vi "Block Profile Measurement v3.vi"() -> ()   [LabVIEW 2011]
uses:
  <vilib>/Utility/error.llb/DialogType.ctl
  <vilib>/DAQmx/read.llb/DAQmx Read (Analog 1D DBL NChan 1Samp).vi
  <vilib>/DAQmx/create/channels.llb/DAQmx Create Channel (AI-Current-Basic).vi
  <vilib>/DAQmx/configure/timing.llb/DAQmx Timing.vi
  <vilib>/DAQmx/configure/trigger.llb/DAQmx Start Trigger (Analog Edge).vi
  <vilib>/DAQmx/miscellaneous.llb/DAQmx Fill In Error Info.vi
  <vilib>/Analysis/NI_AALBase.lvlib
panel:
  in  "Level":dbl=0.5 format="%0.2f"
  in  "Slope":i32(ring)=10280 items=["Rising"=10280, "Falling"=10171]
  in  "Source":string="PFI0" caption="Trigger Source*"
  in  "stop":bool
  out "Measurement":waveform(dbl)[](graph)
  in  "Maximum Value":dbl=10.0 format="%0.2f"
  in  "Minimum Value":dbl=-10.0 format="%0.2f"
  in  "Rate":dbl=50000.0 caption="Sample Rate (Hz)" format="%0.2f"
  in  "Samples per Channel":i32=2048
  in  "Physical Channel":tag="Dev1/ai0"
  out "Scaled Values":dbl[](array[numeric])=[0.0, 1.0] format="%.3p"
  out "Measurements / Block":i32
  in  "ECOLAB Button":bool
  out "Maximum":string="0.000"
  out "Block Count":i32
  in  "Tab Control":enum32{"DISPLAY", "CONFIG", "CALIBRATE"}(tab)
  in  "Intervals":i32=20
  out "XY Graph":cluster{dbl[], "Initialize Value":dbl[]}[](graph)
  out "Histogram Graph":T1(graph)={"X Values"=[0.0, 0.0, 0.0, 0.0, 0.0, 0.0, 0.0, 0.0, 0.0, 0.0, 0.0, 0.0, 0.0, 0.0, 0.0, 0.0, 0.0, 0.0, 0.0, 0.0], "Histogram: h(x)"=[0, 0, 0, 0, 0, 0, 0, 0, 0, 0, 0, 0, 0, 0, 0, 0, 0, 0, 0, 1]}
  in  "Thresh Compare 2":bool=TRUE
  in  "Threshold Value SP 2":dbl=0.004
  in  "Thresh Compare":bool=TRUE
  out "Save Error":errorcluster
  out "Main Error":errorcluster
  out "DAQ Error":errorcluster={"status"=TRUE, "code"=-200478, "source"="Block Profile Measurement v3.vi<append>\n<B>Task Name: </B>mA"}
  in  "DAQ Selection":tag="cDAQ1Mod1/ai0:1"
  in  "Comments (Saves to Data File)":string
  out "DAQ Loop":i32=1641
  out "File Path Output":path=path "H:/Projects/Chris Opelt/Data Files/Data-1-23-2012-{9-AM}.xls"
  in  "Maximum Array Size":i32=200
  in  "Threshold Value SP":dbl=0.004
  in  "DAQ wait ms":u32=1
  in  "Scale":T2={"Channel Select"=0, "Clear/Reset Scales"=FALSE, "Channel #"=["0", "1"], "Scale Names"=["Laser", "Ultra-Sonic"], "Set?"=[FALSE, FALSE, FALSE, FALSE], "HI/LO Setpoints"=[1.0, 0.0, 1.0, 0.0], "Units"=["inches", "inches"], "HI/LO Signals"=[0.02, 0.004, 0.02, 0.004], "Slope/Intercept"=[1.0, 0.0, 1.0, 0.0], "IN/OUT Values"=[0.0, 0.0, 1.0, 1.0], "Sim Signals?"=FALSE, "Sim. Signal"=0.0} {"Sim. Signal" format="%#.3p"; "Channel Select" min=0 step=1; "Slope/Intercept" format="%#.3p"; "HI/LO Setpoints" format="%#.3p"; "IN/OUT Values" format="%#.3p"; "HI/LO Signals" format="%#.3p"}
  in  "Stop Program":bool=TRUE
  in  "Reset Block Count?":bool
  # "Maximum (inches)"
  # "Measurements/Block"
  # "Laser"
  # "Ultrasonic"
  # "Block Count"
  # "Block Profile Measurement Program"
  # "Blake Otting - 2011"
  # "Histogram of Maximum Value Measurements"
  # "Measurement Profile of Last Block"
  # "Laser and Ultrasonic measurements are half-sampled before saving to data row.\nLaser and Ultrasonic measurements are separated by an asterisk in the data row."
  # "Histogram represents laser measurements"
  # "Laser Specs:\nRange:  1.8\" to 2.4\"\nFocal Point:  2.8\"\nResolution:  0.0001\" @ 50mm\nSignal: 4 to 20mA"
  # "These settings should be OK"
  # "Threshold Settings\n(Block Detection & Data Logging Trigger)"
  # "Ultrasonic Specs:\nRange:  1.2\" to 11.8\"\nResolution:  0.025\"\nSignal: 4 to 20mA"
  # "Comparison"
  # "Setpoint (inches)"
  # "LASER"
  # "Comparison"
  # "Setpoint (inches)"
  # "Set to Range (both):\n1.85\" and 2.35\""
  # "ULTRASONIC"
  # "Ch.\n#"
  # "Scale\nName"
  # "Set\nValues?"
  # "Channel\nSelect"
  # "Scaled"
  # "Pre-Scaled"
  # "Scaling Result"
  # "Values"
  # "Units"
  # "Values"
  # "HI"
  # "Slope"
  # "IN"
  # "LO"
  # "Intercept"
  # "OUT"
  # "HI"
  # "Slope"
  # "IN"
  # "LO"
  # "Intercept"
  # "OUT"
  # "HI"
  # "Slope"
  # "IN"
  # "LO"
  # "Intercept"
  # "OUT"
  # "HI"
  # "Slope"
  # "IN"
  # "LO"
  # "Intercept"
  # "OUT"
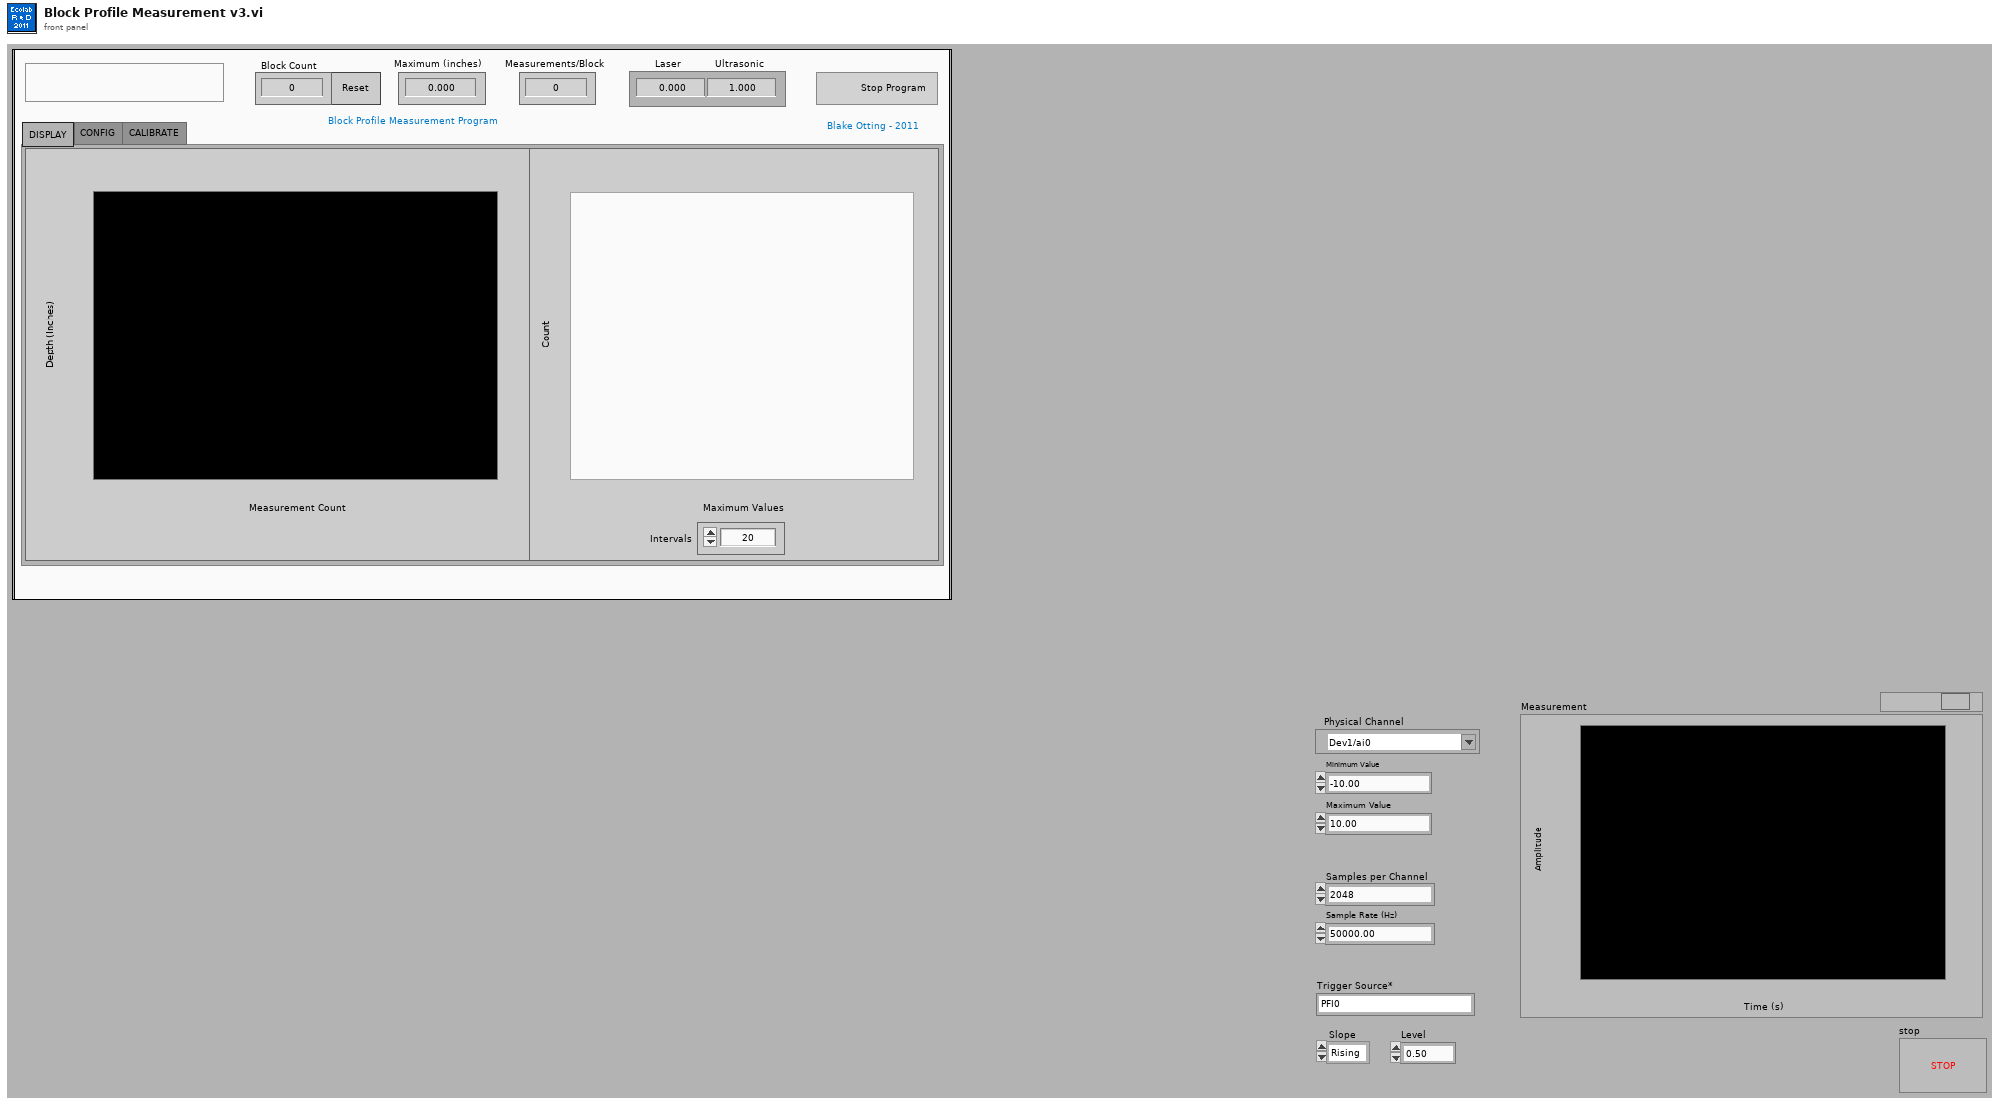
[diagram p1: front panel]
types:
  T1 = cluster{"X Values":dbl[], "Histogram: h(x)":i32[]}
  T2 = cluster{"Channel Select":i32, "Clear/Reset Scales":bool, "Channel #":string[], "Scale Names":string[], "Set?":bool[], "HI/LO Setpoints":dbl[], "Units":string[], "HI/LO Signals":dbl[], "Slope/Intercept":dbl[], "IN/OUT Values":dbl[], "Sim Signals?":bool, "Sim. Signal":dbl}
  T3 = typedef "DialogType.ctl" = u16
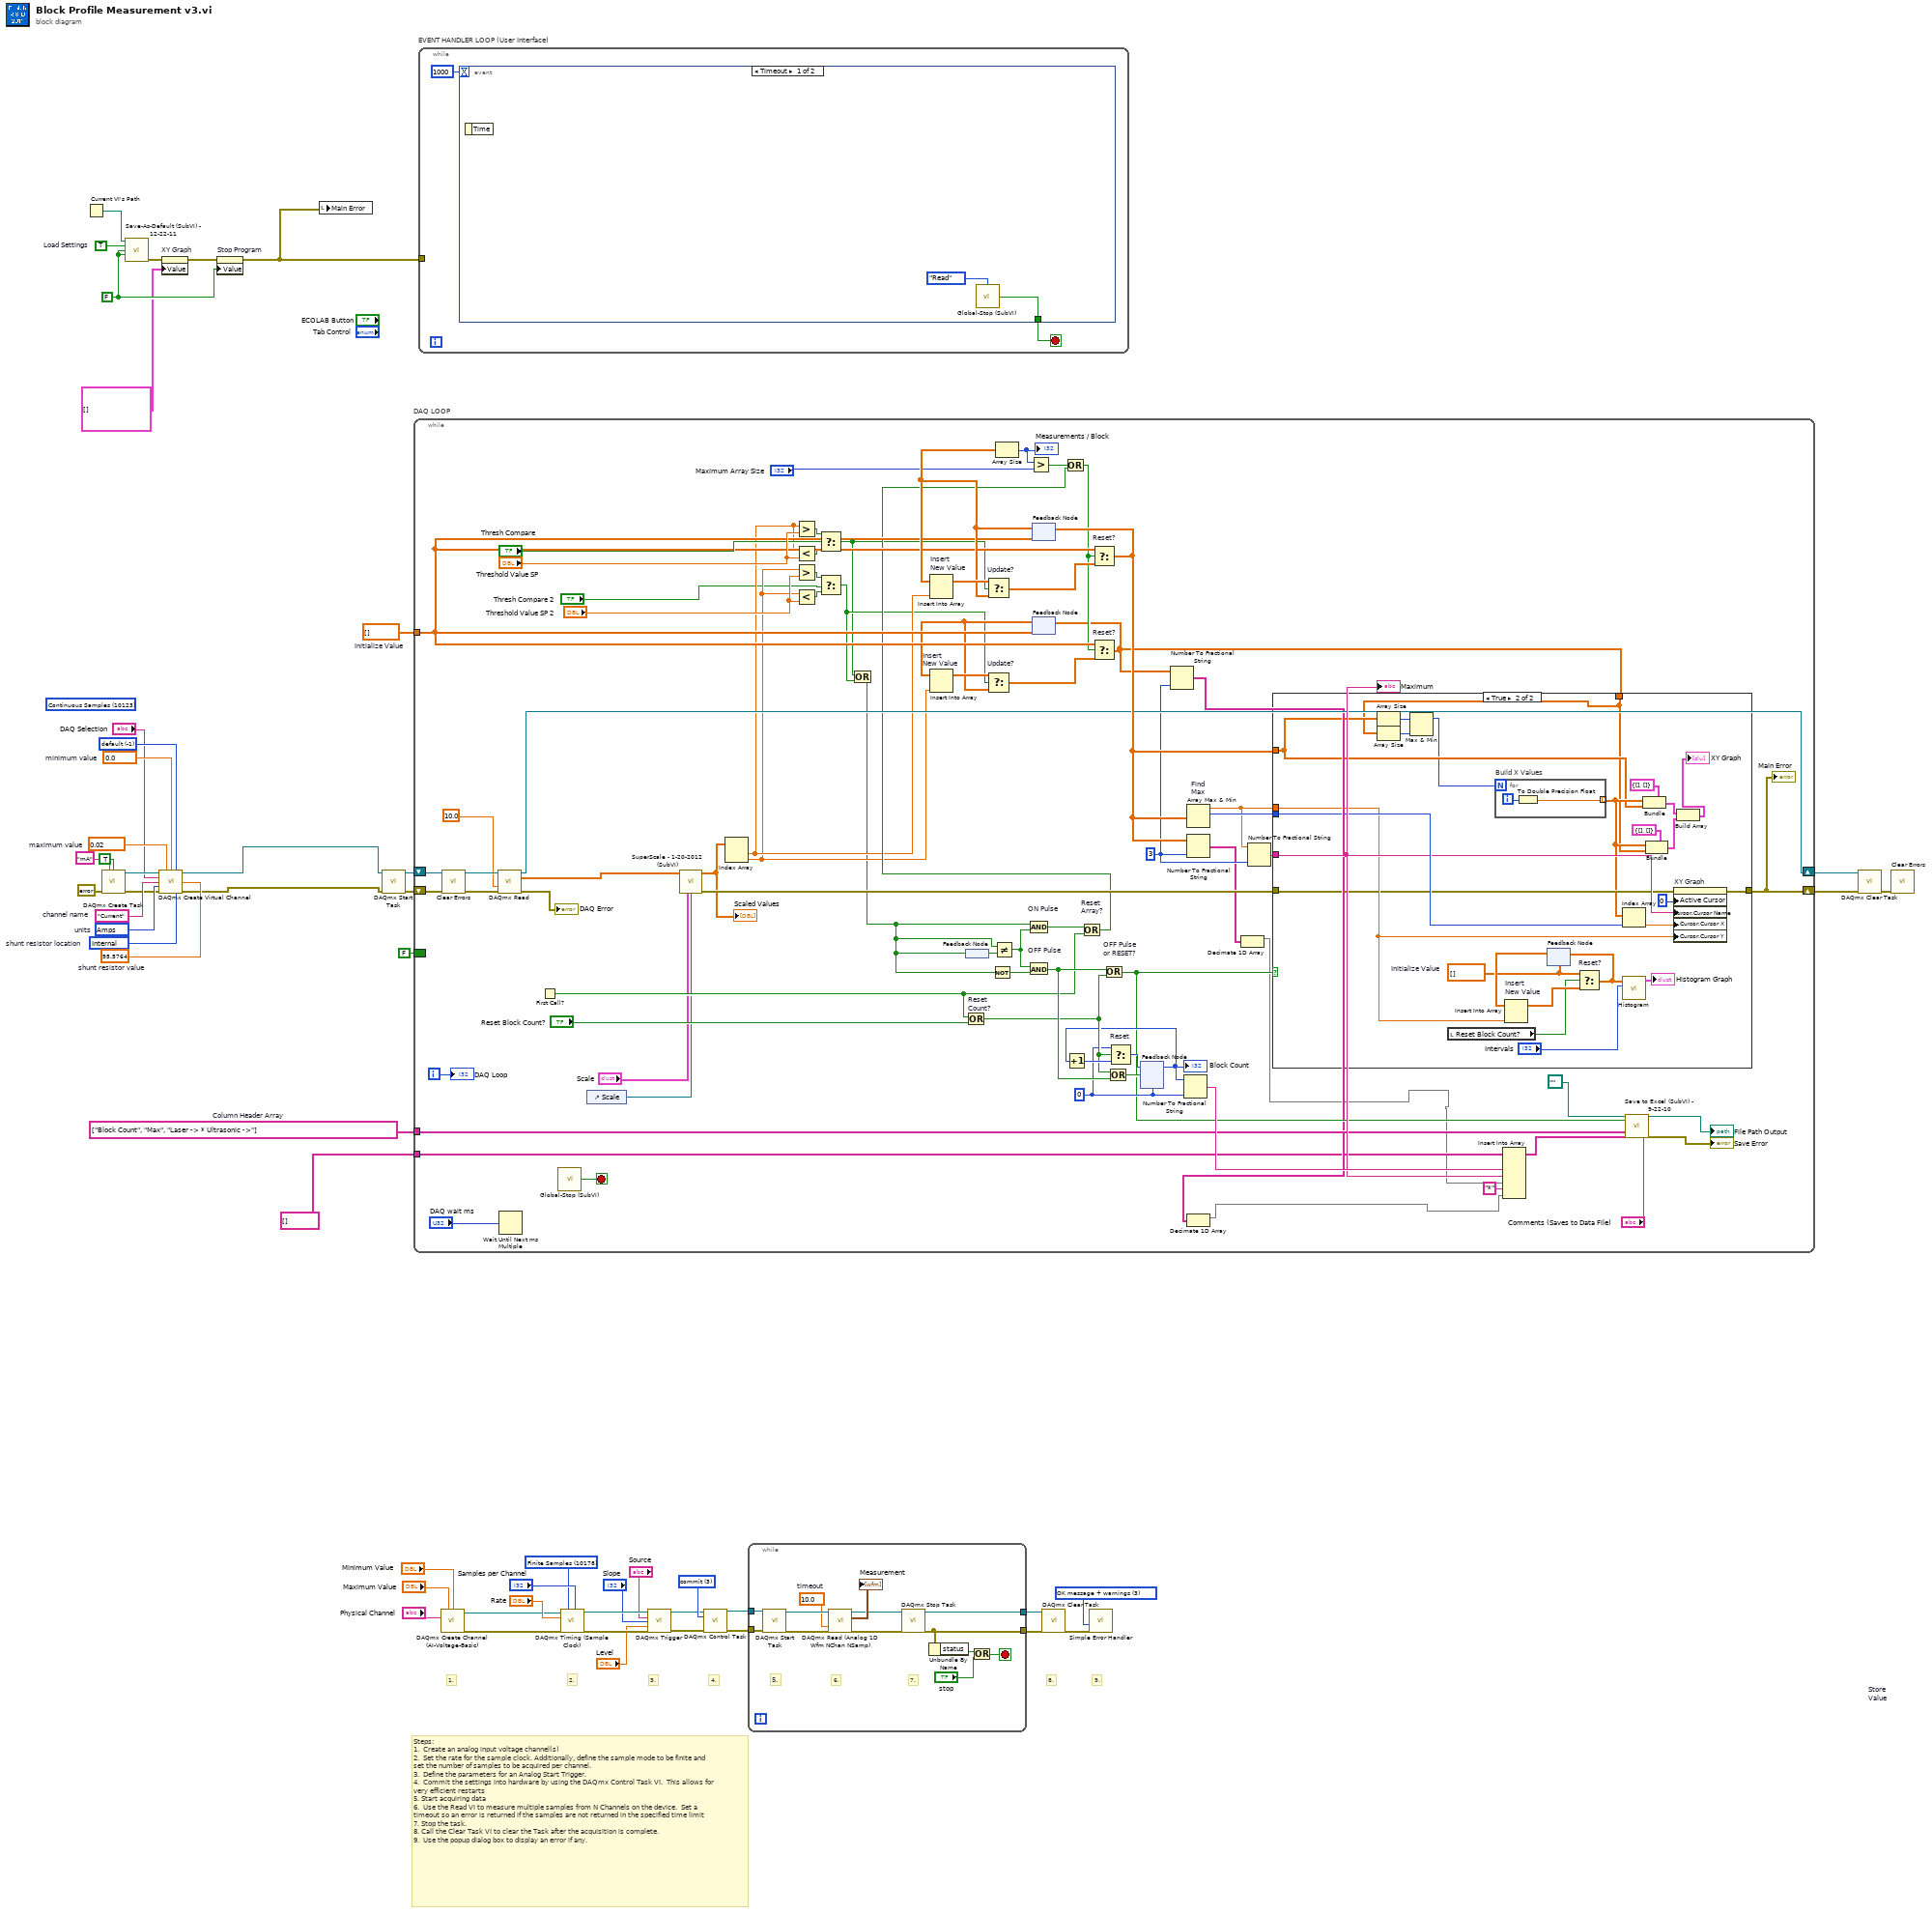
[diagram p0: block diagram]
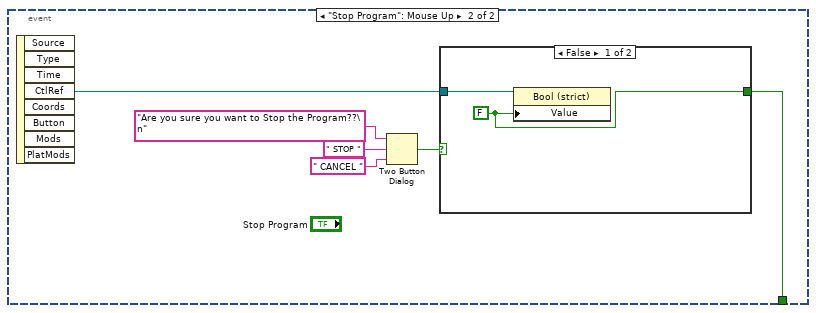
[diagram p2: hidden frame]
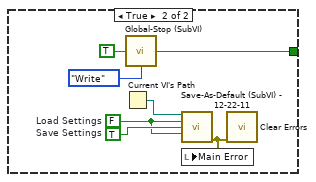
[diagram p3: hidden frame]
diagram:
  w12 = 3 items=["verify"=2, "reserve"=4, "commit"=3, "unreserve"=5, "abort"=6] ("action")
  w13 = T3 3 items=["no dialog", "OK message", "continue or stop message", "OK message + warnings", "continue/stop + warnings"] ("type of dialog (OK msg:1)")
  w14 = 10178 items=["Finite Samples"=10178, "Continuous Samples"=10123] ("sample mode")
  w32 = string[] ["Block Count", "Max", "Laser -> * Ultrasonic ->"]  # Column Header Array
  w34 = dbl[] []  # Initialize Value
  w38 = TRUE  # Load Settings
  w37 = FALSE
  (unwired) 10123 items=["Finite Samples"=10178, "Continuous Samples"=10123, "Hardware Timed Single Point"=12522] ("Sample Mode")
  w46 = -1 items=["default"=-1, "RSE"=10083, "NRSE"=10078, "Differential"=10106, "Pseudodifferential"=12529]
  w47 = 10342 items=["Amps"=10342, "From Custom Scale"=10065]  # units
  w48 = 95.5764  # shunt resistor value
  w49 = 10200 items=["Internal"=10200, "External"=10167]  # shunt resistor location
  w50 = "Current"  # channel name
  w51 = 0.0  # minimum value
  w52 = 0.02  # maximum value
  # "9."
  # "8."
  # "4."
  # "Steps: \n1.  Create an analog input voltage channel(s)\n2.  Set the rate for the sample clock. Additionally, define the sample mode to be finite and set the number of samples to be acquired per channel.\n3.  Define the parameters for an Analog Start Trigger.\n4.  Commit the settings into hardware by using the DAQmx Control Task VI.  This allows for very efficient restarts\n5. Start acquiring data\n6.  Use the Read VI to measure multiple samples from N Channels on the device.  Set a timeout so an error is returned if the samples are not returned in the specified time limit\n7. Stop the task.\n8. Call the Clear Task VI to clear the Task after the acquisition is complete.\n9.  Use the popup dialog box to display an error if any."
  # "3."
  # "2."
  # "1."
  n1 = Current VI's Path() -> (path=w39:path)
  n2 = call <vilib>:"DAQmx Create Task.vi"("new task name"="mA", "auto cleanup"=TRUE, "error in"=errorcluster {"status"=FALSE, "code"=0, "source"=""}) -> ("task out"=w45:refnum<k21>, "error out"=w44:errorcluster)  [unwired: 11 in]
  n3 = call "Save-As-Default (SubVI) - 12-22-11.vi"("Current VI's Path"=w39, "Load Settings"=w38, "Save Settings"=w37, "Save and Exit"=w37) -> ("Error Output"=w36:errorcluster)  [unwired: 11 in]
  n4 = call-poly <vilib>:"DAQmx Create Virtual Channel.vi"("task in"=w45, "maximum value"=w52, "minimum value"=w51, "input terminal configuration"=w46, "physical channels"="DAQ Selection", "name to assign"=w50, "external shunt resistor value"=w48, "units"=w47, "error in"=w44, "shunt resistor location"=w49) -> ("task out"=w24:refnum<k21>, "error out"=w23:errorcluster)  [unwired: 1 in, 3 out]
  n5 = property on="XY Graph" class="XYGraph (strict)"(error in=w36, "Value"=cluster{dbl[], "Initialize Value":dbl[]}[] [] ("XY Graph")) -> (error out=w35:errorcluster)  [unwired: 1 in, 1 out]
  n6 = property on="Stop Program" class="Bool (strict)"(error in=w35, "Value"=w37) -> (error out=w33:errorcluster)  [unwired: 1 in, 1 out]
  n7 = local write "Main Error"(w33) -> ()
  n8 = call <vilib>:"DAQmx Start Task.vi"("task/channels in"=w24, "error in"=w23) -> ("task out"=w29:refnum<k21>, "error out"=w27:errorcluster)  [unwired: 12 in]
  n9 = while "DAQ LOOP" {
    tunnel: w34 -> [w82]
    tunnel: w32 -> [w102]
    tunnel: string[] [] ("F-format string") -> [w76]
    shift-right: [w94] -> w28
    shift-left: w29 -> [w90]
    shift-right: [w97] -> w40
    shift-left: w27 -> [w91]
    border: FALSE -> [_]
    i -> [w126]
    stop <- w124 stop-if-true
    w79 = i16 3 ("precision (6)")
    w99 = 0 ("index")
    n10 = call <vilib>:"Clear Errors.vi"("error in (no error)"=w91) -> ("error out"=w89:errorcluster)  [unwired: 6 in]
    n11 = call-poly <vilib>:"DAQmx Read.vi"("task/channels in"=w90, "timeout"=10.0, "error in"=w89) -> ("task out"=w94:refnum<k21>, "data"=w54:dbl[], "error out"=→"DAQ Error":errorcluster)  [unwired: 10 in]
    n12 = Wait Until Next ms Multiple(millisecond multiple="DAQ wait ms") -> ()  [unwired: 1 out]
    n13 = First Call?() -> (First Call?: T/F=w100:bool)
    n14 = call "Global-Stop (SubVI).vi"() -> ("OUT"=w124:bool)  [unwired: 4 in]
    n15 = control-ref of="Scale"() -> (w69:refnum<vi>)
    n16 = call "SuperScale - 1-20-2012 (SubVI).vi"("Measured Signals"=w54, "Scale Template"="Scale", "Scale Reference"=w69) -> ("Scaled Values"=w66:dbl[], "Scale Error"=w98:errorcluster)  [unwired: 11 in]
    "Scaled Values" <- w66
    n17 = Index Array(array=w66) -> (element #1=w61:dbl, element #2=w60:dbl)  [unwired: 2 in]
    n18 = Greater?(x=w61, y="Threshold Value SP") -> (0:w68:bool)
    n19 = Less?(x=w61, y="Threshold Value SP") -> (x < y?=w67:bool)
    n20 = Greater?(x=w60, y="Threshold Value SP 2") -> (0:w64:bool)
    n21 = Less?(x=w60, y="Threshold Value SP 2") -> (x < y?=w63:bool)
    n22 = Select(t=w68, s="Thresh Compare", f=w67) -> (s? t:f=w57:bool)
    n23 = Select(t=w64, s="Thresh Compare 2", f=w63) -> (s? t:f=w58:bool)
    n24 = Or(x=w57, y=w58) -> (x .or. y?=w56:bool)
    n25 = Or "Reset\nCount?"(x=w100, y="Reset Block Count?") -> (x .or. y?=w114:bool)
    n26 = feedback #1() -> (w121:bool)
    n27 = feedback-in #1(w56) -> ()
    n28 = Not(x=w56) -> (.not. x?=w119:bool)
    n29 = Not Equal?(x=w56, y=w121) -> (x != y?=w120:bool)
    n30 = And "ON Pulse"(x=w56, y=w120) -> (x .and. y?=w101:bool)
    n31 = And "OFF Pulse"(x=w120, y=w119) -> (x .and. y?=w115:bool)
    n32 = feedback #2(w82) -> (w88:dbl[])
    n33 = Insert Into Array "Insert \nNew Value"(array=w88, new element=w61) -> (w123:dbl[])  [unwired: 1 in]
    n34 = Select "Update?"(t=w123, s=w57, f=w88) -> (s? t:f=w122:dbl[])
    n35 = Array Size(array=w88) -> (size(s)=w87:i32)
    "Measurements / Block" <- w87
    n36 = Greater?(x=w87, y="Maximum Array Size") -> (0:w85:bool)
    n37 = feedback #3(w82) -> (w80:dbl[])
    n38 = Insert Into Array "Insert \nNew Value"(array=w80, new element=w60) -> (w84:dbl[])  [unwired: 1 in]
    n39 = Select "Update?"(t=w84, s=w58, f=w80) -> (s? t:f=w83:dbl[])
    n40 = Or "Reset\nArray?"(x=w101, y=w100) -> (x .or. y?=w72:bool)
    n41 = Or(x=w85, y=w72) -> (x .or. y?=w81:bool)
    n42 = Select "Reset?"(t=w82, s=w81, f=w122) -> (s? t:f=w103:dbl[])
    n43 = feedback-in #2(w103) -> ()
    n44 = Select "Reset?"(t=w82, s=w81, f=w83) -> (s? t:f=w71:dbl[])
    n45 = feedback-in #3(w71) -> ()
    n46 = Or "OFF Pulse\nor RESET?"(x=w115, y=w114) -> (x .or. y?=w95:bool)
    n47 = Or(x=w114, y=w115) -> (x .or. y?=w116:bool)
    n48 = feedback #4 "Store\nValue"(w99) -> (w107:i32)
    "Block Count" <- w107
    n49 = Increment(x=w107) -> (x+1=w118:i32)
    n50 = Select "Reset"(t=w99, s=w114, f=w118) -> (s? t:f=w117:i32)
    n51 = feedback-in #4(w117, w116) -> ()
    n52 = Number To Fractional String(number=w71, precision (6)=w79) -> (F-format string=w78:string[])  [unwired: 2 in]
    n53 = Number To Fractional String(number=w107, precision (6)=w99) -> (F-format string=w112:string)  [unwired: 2 in]
    n54 = Decimate 1D Array(w78) -> (w73:string[])  [unwired: 1 out]
    n55 = Array Max & Min "Find\nMax"(array=w103) -> (max value=w105:dbl, max index (indices)=w106:i32)  [unwired: 2 out]
    n56 = Number To Fractional String(number=w103, precision (6)=w79) -> (F-format string=w77:string[])  [unwired: 2 in]
    n57 = Decimate 1D Array(w77) -> (w74:string[])  [unwired: 1 out]
    n58 = Number To Fractional String(number=w105, precision (6)=w79) -> (F-format string=w104:string)  [unwired: 2 in]
    "Maximum" <- w104
    n59 = case shown="True" w95 {
      tunnel: w103 -> [_ w132]
      tunnel: w106 -> [_ w144]
      tunnel: w104 -> [_ w143]
      tunnel: w105 -> [_ w142]
      tunnel: w98 -> [w127 w139]
      tunnel: [w127 w138] -> w97
      tunnel: w71 -> [_ w130]
      frame False {
      }
      frame True {
        w151 = dbl[] []  # Initialize Value
        n60 = Array Size(array=w132) -> (size(s)=w131:i32)
        n61 = Array Size(array=w130) -> (size(s)=w129:i32)
        n62 = Max & Min(x=w131, y=w129) -> (max(x,y)=w128:i32)  [unwired: 1 out]
        n63 = local read "Reset Block Count?"() -> (w140:bool)
        n64 = for "Build X Values" {
          N: w128 -> [_]
          tunnel: [w153] -> w136 mode=indexing
          i -> [w154]
          n65 = To Double Precision Float(number=w154) -> (double precision float=w153:dbl)
        }
        n66 = feedback #5(w151) -> (w152:dbl[])
        n67 = Insert Into Array "Insert \nNew Value"(array=w152, new element=w142) -> (w141:dbl[])  [unwired: 1 in]
        n68 = Select "Reset?"(t=w151, s=w140, f=w141) -> (s? t:f=w150:dbl[])
        n69 = feedback-in #5(w150) -> ()
        n70 = call <vilib>:"Histogram.vi"("intervals"="Intervals", "X"=w150) -> ("Histogram Graph"=→"Histogram Graph":T1)  [unwired: 6 in, 3 out]
        n71 = Index Array(array=w136, index=w144) -> (element=w146:dbl)
        n72 = Bundle(cluster=cluster{dbl[], "Initialize Value":dbl[]} {[], "Initialize Value"=[]}, w136, "Initialize Value"=w132) -> (w135:cluster{dbl[], "Initialize Value":dbl[]})
        n73 = Bundle(cluster=cluster{dbl[], "Initialize Value":dbl[]} {[], "Initialize Value"=[]}, w136, "Initialize Value"=w130) -> (w134:cluster{dbl[], "Initialize Value":dbl[]})
        n74 = property on="XY Graph" class="XYGraph (strict)"(error in=w139, "Active Cursor"=u32 0, "Cursor.Cursor Name"=w143, "Cursor.Cursor X"=w146, "Cursor.Cursor Y"=w142) -> (error out=w138:errorcluster)  [unwired: 1 in, 1 out]
        n75 = Build Array(w135, w134) -> (→"XY Graph":cluster{dbl[], "Initialize Value":dbl[]}[])
      }
    }
    "Main Error" <- w97
    n76 = Insert Into Array(array=w76, new element #1=w112, new element #2=w104, new element #3=w74, new element #4="*" ("new element/subarray"), new element #5=w73) -> (w111:string[])  [unwired: 1 in]
    n77 = call "Save to Excel (SubVI) - 9-22-10.vi"("File Path Input"=path "", "Save (Enable/Signal)"=w95, "Column Header Array"=w102, "Data Array (Row)"=w111, "Comments"="Comments (Saves to Data File)") -> ("File Path Output"=→"File Path Output":path, "Error Output"=→"Save Error":errorcluster)  [unwired: 10 in, 3 out]
    "DAQ Loop" <- w126
  }
  n78 = while "EVENT HANDLER LOOP (User Interface)" {
    tunnel: w33 -> [_]
    stop <- w156 stop-if-true
    n79 = event shown="[0] Timeout" {
      selector: _ -> [_ _]
      dyn-events: _ -> [_ _]
      timeout: 1000 -> [_ _]
      tunnel: [w157 w160] -> w156
      event Timeout {
        n80 = event-data() -> ()  [unwired: 2 out]
        n81 = call "Global-Stop (SubVI).vi"("Mode (Read)"=enum16{"Read", "Write"}."Read") -> ("OUT"=w157:bool)  [unwired: 3 in]
      }
      event "Stop Program": Mouse Up {
        n82 = event-data() -> ("CtlRef"=w159:refnum<vi>)  [unwired: 8 out]
        n83 = Two Button Dialog(message="Are you sure you want to Stop the Program??\n", 1:" CANCEL " ("F button name (\"Cancel\")"), 2:" STOP ") -> (T button?=w161:bool)
        n84 = case shown="False" w161 {
          tunnel: [w165 w171] -> w160
          tunnel: w159 -> [w166 _]
          frame False {
            w165 = FALSE ("Value")
            n85 = property class="Bool (strict)"(reference=w166, "Value"=w165) -> ()  [unwired: 1 in, 2 out]
          }
          frame True {
            w169 = TRUE  # Save Settings
            w168 = FALSE  # Load Settings
            n86 = Current VI's Path() -> (path=w170:path)
            n87 = call "Global-Stop (SubVI).vi"("Mode (Read)"=enum16{"Read", "Write"}."Write", "IN"=TRUE) -> ("OUT"=w171:bool)  [unwired: 2 in]
            n88 = call "Save-As-Default (SubVI) - 12-22-11.vi"("Current VI's Path"=w170, "Load Settings"=w168, "Save Settings"=w169, "Save and Exit"=w168) -> ("Error Output"=w167:errorcluster)  [unwired: 11 in]
            n89 = local write "Main Error"(w167) -> ()
            n90 = call <vilib>:"Clear Errors.vi"("error in (no error)"=w167) -> ()  [unwired: 7 out]
          }
        }
      }
    }
  }
  n91 = call-poly <vilib>:"DAQmx Create Channel (AI-Voltage-Basic).vi"("maximum value"="Maximum Value", "minimum value"="Minimum Value", "physical channels"="Physical Channel") -> ("task out"=w16:refnum<k21>, "error out"=w20:errorcluster)  [unwired: 11 in]
  n92 = call-poly <vilib>:"DAQmx Timing (Sample Clock).vi"("task/channels in"=w16, "sample mode"=w14, "samples per channel"="Samples per Channel", "rate"="Rate", "error in"=w20) -> ("task out"=w7:refnum<k21>, "error out"=w6:errorcluster)  [unwired: 9 in]
  n93 = call-poly <vilib>:"DAQmx Trigger.vi"("task/channels in"=w7, "source"="Source", "slope"="Slope", "level"="Level", "error in"=w6) -> ("task out"=w5:refnum<k21>, "error out"=w4:errorcluster)  [unwired: 9 in]
  n94 = call <vilib>:"DAQmx Control Task.vi"("task/channels in"=w5, "action"=w12, "error in"=w4) -> ("task out"=w11:refnum<k21>, "error out"=w10:errorcluster)  [unwired: 11 in]
  n95 = while {
    tunnel: w11 -> [w186]
    tunnel: w10 -> [w185]
    tunnel: [w184] -> w9
    tunnel: [w177] -> w8
    stop <- w174 stop-if-true
    w180 = 10.0  # timeout
    # "7."
    # "6."
    # "5."
    n96 = call <vilib>:"DAQmx Start Task.vi"("task/channels in"=w186, "error in"=w185) -> ("task out"=w182:refnum<k21>, "error out"=w183:errorcluster)  [unwired: 12 in]
    n97 = call-poly <vilib>:"DAQmx Read (Analog 1D Wfm NChan NSamp).vi"("task/channels in"=w182, "timeout"=w180, "error in"=w183) -> ("task out"=w179:refnum<k21>, "data"=→"Measurement":waveform(dbl)[], "error out"=w178:errorcluster)  [unwired: 10 in]
    n98 = call <vilib>:"DAQmx Stop Task.vi"("task/channels in"=w179, "error in"=w178) -> ("task out"=w184:refnum<k21>, "error out"=w177:errorcluster)  [unwired: 12 in]
    n99 = Unbundle By Name(w177) -> ("status"=w176:bool)
    n100 = Or(x=w176, y="stop") -> (x .or. y?=w174:bool)
  }
  n101 = call <vilib>:"DAQmx Clear Task.vi"("task in"=w9, "error in"=w8) -> ("error out"=w18:errorcluster)  [unwired: 13 in]
  n102 = call <vilib>:"Simple Error Handler.vi"("type of dialog (OK msg:1)"=w13, "error in (no error)"=w18) -> ()  [unwired: 3 in, 5 out]
  n103 = call <vilib>:"DAQmx Clear Task.vi"("task in"=w28, "error in"=w40) -> ("error out"=w53:errorcluster)  [unwired: 13 out]
  n104 = call <vilib>:"Clear Errors.vi"("error in (no error)"=w53) -> ()  [unwired: 6 in, 1 out]
